vi "LINC Handshake Global.vi"(5 "target name":string, 7 "mode":T4, 8 "error in (no error)":errorcluster, 9 "handshake in":T1, 10 "command in":T2, 11 "GUID":string) -> (0 "error out":errorcluster, 1 "handshake out":T1, 2 "command out":T2, 3 "handshake":bool)   [LabVIEW 2018, in "STEPkgDriver_LINC.lvlib"]
uses:
  STEPkgDriver_LINC.lvlib
  LINC Command Origin.ctl
  LINC Command.ctl
  LINC Handshake Internal.ctl
  LINC Global Handshake Mode.ctl
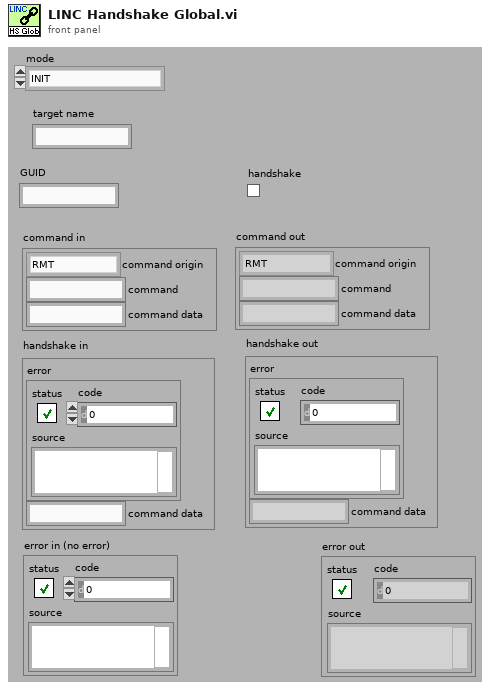
[diagram p1: front panel]
types:
  T1 = typedef "STEPkgDriver_LINC.lvlib/LINC Handshake Internal.ctl" = cluster{"error":errorcluster, "command data":string}
  T2 = typedef "STEPkgDriver_LINC.lvlib/LINC Command.ctl" = cluster{"command origin":T3, "command":string, "command data":string}
  T3 = typedef "STEPkgDriver_LINC.lvlib/LINC Command Origin.ctl" = enum8{"RMT", "LCL"}
  T4 = typedef "STEPkgDriver_LINC.lvlib/LINC Global Handshake Mode.ctl" = enum16{"INIT", "CLEAR", "ADD_COMMAND", "RMV_COMMAND", "CLR_HANDSHAKE", "SET_HANDSHAKE", "GET_HANDSHAKE"}
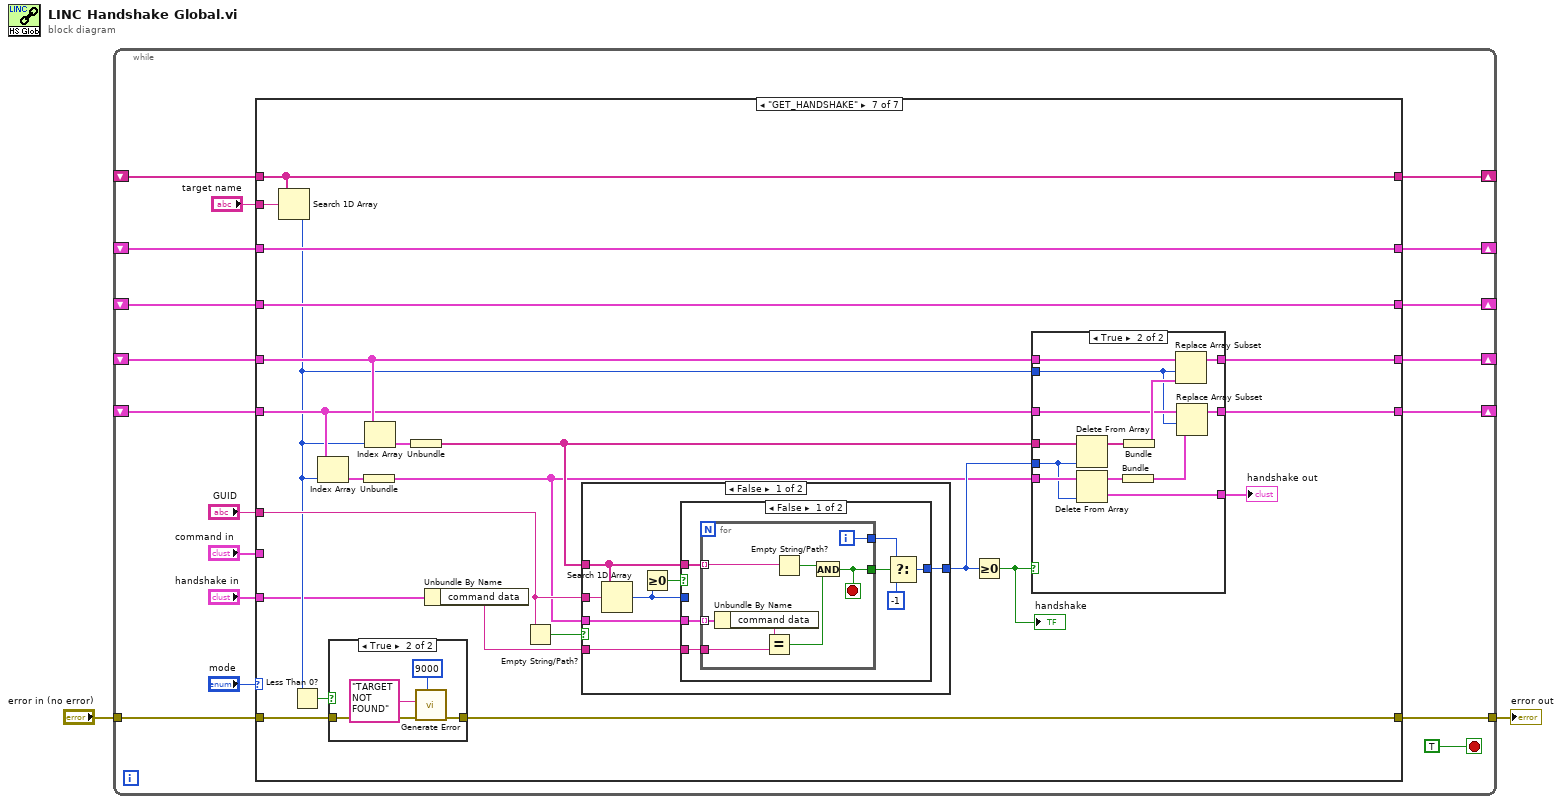
[diagram p0: block diagram]
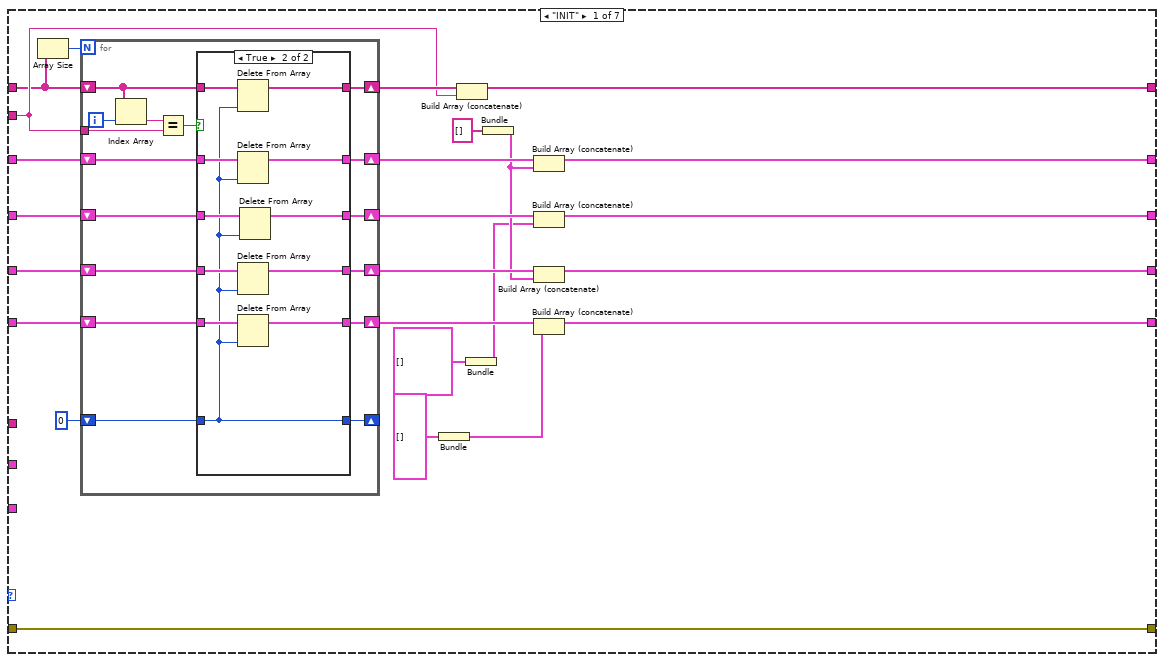
[diagram p2: hidden frame]
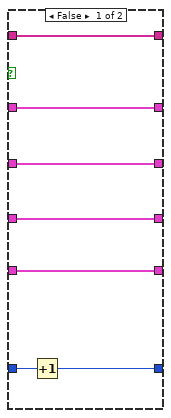
[diagram p3: hidden frame]
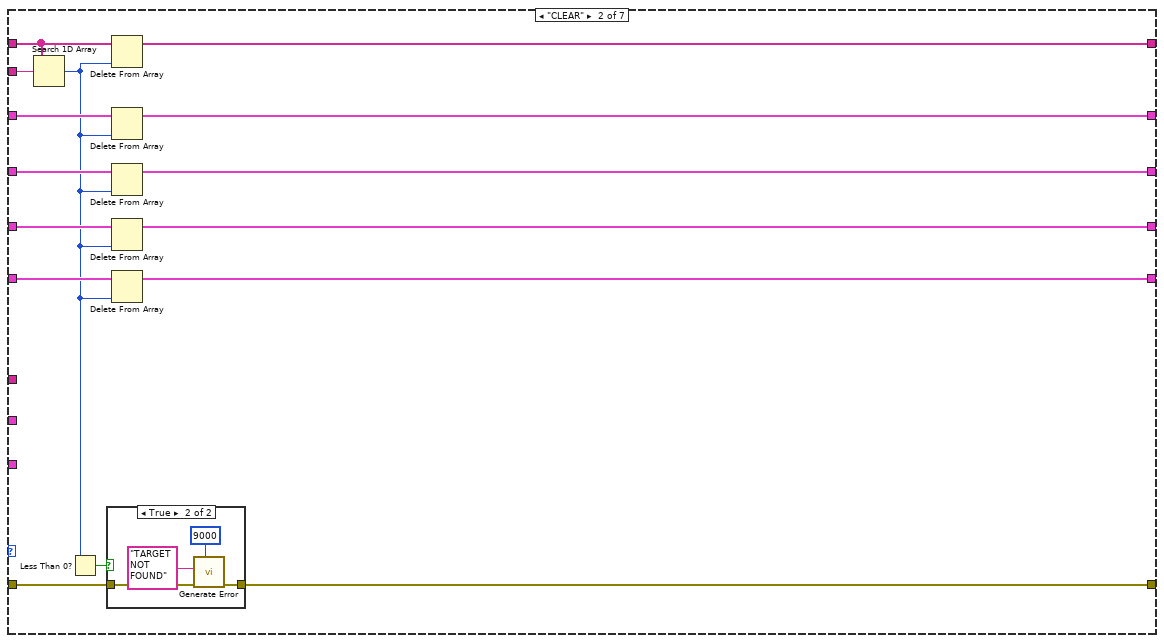
[diagram p4: hidden frame]
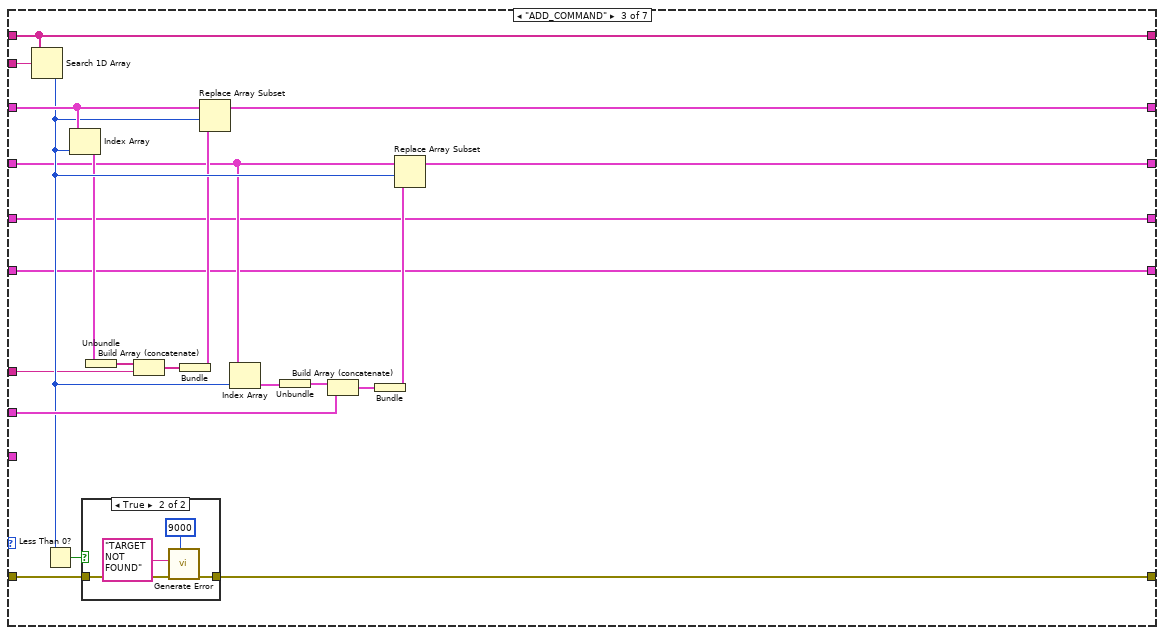
[diagram p6: hidden frame]
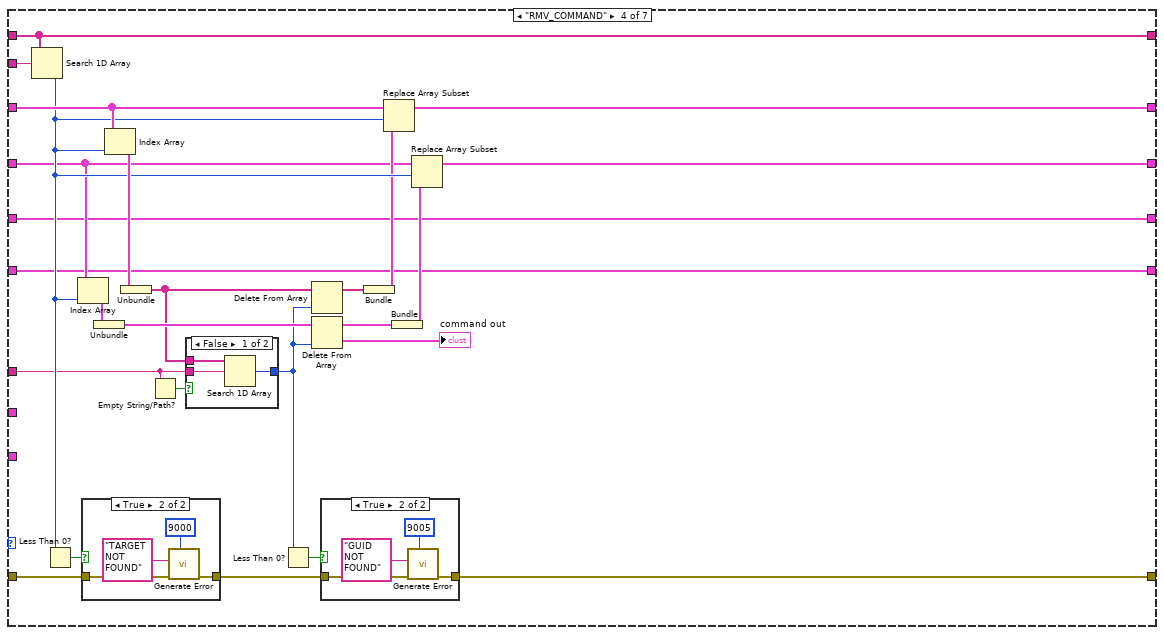
[diagram p8: hidden frame]
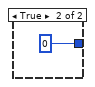
[diagram p9: hidden frame]
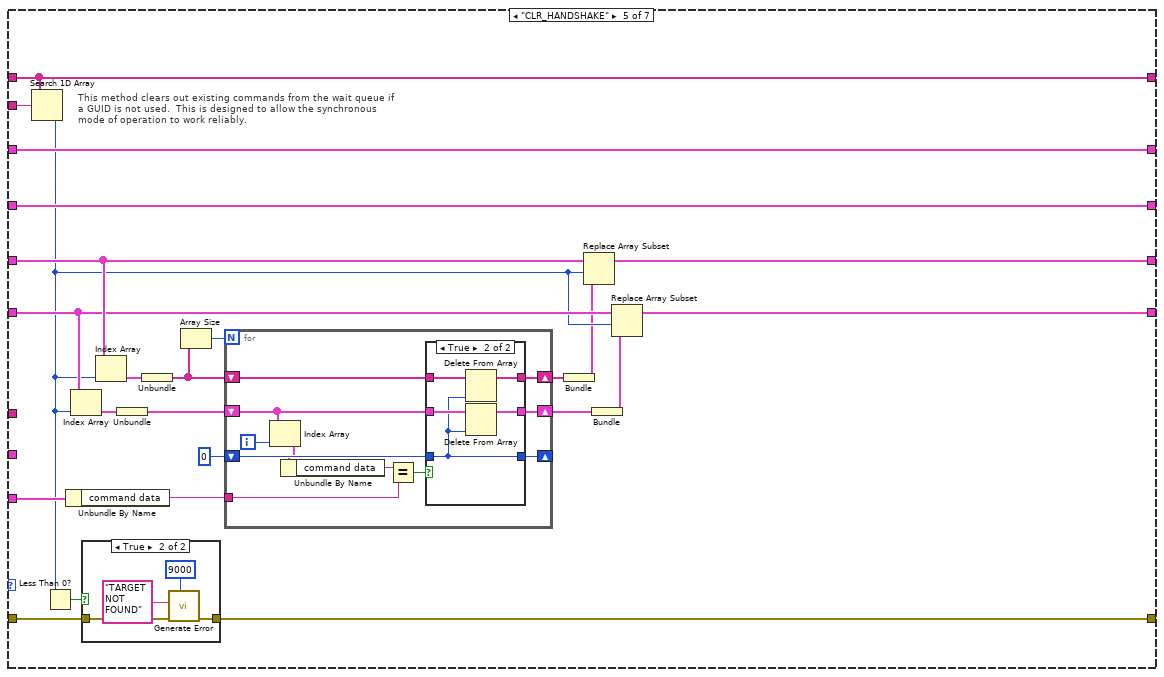
[diagram p12: hidden frame]
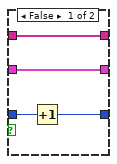
[diagram p13: hidden frame]
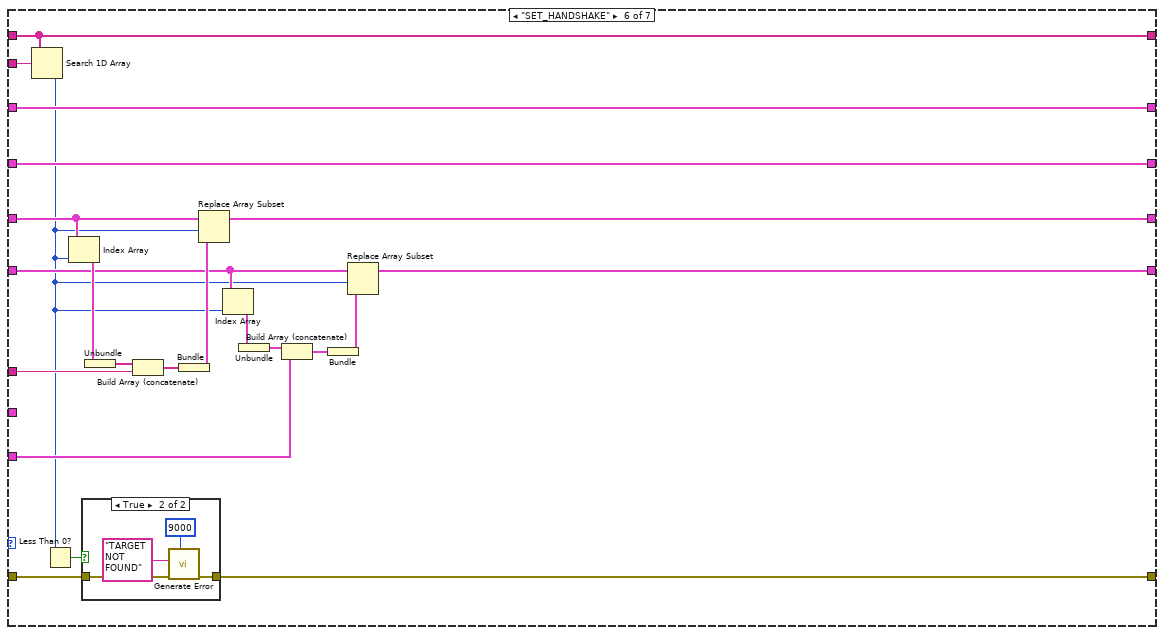
[diagram p15: hidden frame]
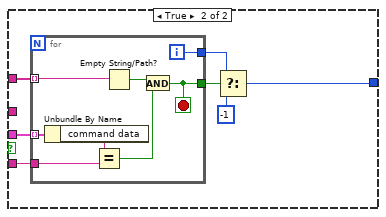
[diagram p19: hidden frame]
diagram:
  n1 = while {
    shift-right: [w18] -> _
    shift-left: _ -> [w19]
    tunnel: "error in (no error)" -> [w15]
    tunnel: [w14] -> w1
    shift-right: [w12] -> _
    shift-left: _ -> [w13]
    shift-right: [w10] -> _
    shift-left: _ -> [w9]
    shift-right: [w7] -> _
    shift-left: _ -> [w6]
    shift-right: [w5] -> _
    shift-left: _ -> [w4]
    stop <- TRUE stop-if-true
    n2 = case shown="\"GET_HANDSHAKE\"" "mode" {
      tunnel: w19 -> [w39 w93 w120 w151 w189 w236 w264]
      tunnel: [w45 w92 w120 w151 w189 w236 w264] -> w18
      tunnel: "target name" -> [w40 w94 w121 w152 w190 w237 w265]
      tunnel: w15 -> [w44 w90 w118 w149 w188 w234 w262]
      tunnel: [w44 w89 w117 w136 w186 w233 w256] -> w14
      tunnel: w13 -> [w41 w88 w101 w129 w184 w226 w252]
      tunnel: [w43 w87 w101 w129 w183 w225 w251] -> w12
      tunnel: "command in" -> [_ _ w114 _ _ _ _]
      tunnel: [w33 w85 w111 w147 w187 w227 w257] -> w10
      tunnel: w9 -> [w31 w86 w110 w148 w187 w227 w257]
      tunnel: "GUID" -> [_ _ w104 w133 _ w228 w259]
      tunnel: [w30 w83 w102 w131 w185 w224 w253] -> w7
      tunnel: w6 -> [w29 w84 w103 w130 w185 w224 w253]
      tunnel: w4 -> [w26 w82 w100 w128 w181 w222 w249]
      tunnel: [w25 w80 w100 w128 w182 w223 w250] -> w5
      tunnel: "handshake in" -> [_ _ _ _ w180 w217 w245]
      frame "INIT" {
        n3 = Array Size(array=w39) -> (size(s)=w38:i32)
        n4 = for {
          N: w38 -> [_]
          shift-right: [w55] -> w42
          shift-left: w39 -> [w60]
          shift-right: [w54] -> w36
          shift-left: w41 -> [w59]
          tunnel: w40 -> [w57]
          shift-right: [w52] -> _
          shift-left: 0 -> [w53]
          shift-right: [w50] -> w32
          shift-left: w31 -> [w51]
          shift-right: [w48] -> w28
          shift-left: w29 -> [w49]
          shift-right: [w47] -> w27
          shift-left: w26 -> [w46]
          i -> [w61]
          n5 = Index Array(array=w60, index=w61) -> (element=w58:string)
          n6 = Equal?(x=w58, y=w57) -> (x = y?=w56:bool)
          n7 = case shown="True" w56 {
            tunnel: w60 -> [w68 w79]
            tunnel: w59 -> [w67 w77]
            tunnel: [w68 w78] -> w55
            tunnel: [w67 w76] -> w54
            tunnel: w53 -> [w66 w69]
            tunnel: [w65 w69] -> w52
            tunnel: w51 -> [w64 w75]
            tunnel: [w64 w74] -> w50
            tunnel: w49 -> [w63 w73]
            tunnel: [w63 w72] -> w48
            tunnel: w46 -> [w62 w70]
            tunnel: [w62 w71] -> w47
            frame False {
              n8 = Increment(x=w66) -> (x+1=w65:i32)
            }
            frame True {
              n9 = Delete From Array(array=w79, index=w69) -> (array with subset deleted=w78:string[])  [unwired: 1 in, 1 out]
              n10 = Delete From Array(array=w75, index=w69) -> (array with subset deleted=w74:cluster{string[]}[])  [unwired: 1 in, 1 out]
              n11 = Delete From Array(array=w77, index=w69) -> (array with subset deleted=w76:cluster{string[]}[])  [unwired: 1 in, 1 out]
              n12 = Delete From Array(array=w70, index=w69) -> (array with subset deleted=w71:cluster{T1[]}[])  [unwired: 1 in, 1 out]
              n13 = Delete From Array(array=w73, index=w69) -> (array with subset deleted=w72:cluster{T2[]}[])  [unwired: 1 in, 1 out]
            }
          }
        }
        n14 = Bundle(T1[] []) -> (w21:cluster{T1[]})  [unwired: 1 in]
        n15 = Build Array (concatenate)(w42, w40) -> (w45:string[])
        n16 = Bundle(T2[] []) -> (w23:cluster{T2[]})  [unwired: 1 in]
        n17 = Bundle(string[] []) -> (w24:cluster{string[]})  [unwired: 1 in]
        n18 = Build Array (concatenate)(w32, w24) -> (w33:cluster{string[]}[])
        n19 = Build Array (concatenate)(w28, w23) -> (w30:cluster{T2[]}[])
        n20 = Build Array (concatenate)(w36, w24) -> (w43:cluster{string[]}[])
        n21 = Build Array (concatenate)(w27, w21) -> (w25:cluster{T1[]}[])
      }
      frame "CLEAR" {
        n22 = Search 1D Array(1D array=w93, element=w94) -> (index of element=w81:i32)  [unwired: 1 in]
        n23 = Less Than 0?(x=w81) -> (x < 0?=w91:bool)
        n24 = case shown="True" w91 {
          tunnel: w90 -> [w95 w99]
          tunnel: [w95 w98] -> w89
          frame False {
          }
          frame True {
            n25 = call "Generate Error.vi"("error code (-1301)"=9000, "error in"=w99, "description"="TARGET NOT FOUND") -> ("error out"=w98:errorcluster)  [unwired: 8 in]
          }
        }
        n26 = Delete From Array(array=w93, index=w81) -> (array with subset deleted=w92:string[])  [unwired: 1 in, 1 out]
        n27 = Delete From Array(array=w86, index=w81) -> (array with subset deleted=w85:cluster{string[]}[])  [unwired: 1 in, 1 out]
        n28 = Delete From Array(array=w84, index=w81) -> (array with subset deleted=w83:cluster{T2[]}[])  [unwired: 1 in, 1 out]
        n29 = Delete From Array(array=w88, index=w81) -> (array with subset deleted=w87:cluster{string[]}[])  [unwired: 1 in, 1 out]
        n30 = Delete From Array(array=w82, index=w81) -> (array with subset deleted=w80:cluster{T1[]}[])  [unwired: 1 in, 1 out]
      }
      frame "ADD_COMMAND" {
        n31 = Search 1D Array(1D array=w120, element=w121) -> (index of element=w109:i32)  [unwired: 1 in]
        n32 = Less Than 0?(x=w109) -> (x < 0?=w119:bool)
        n33 = Index Array(array=w110, index=w109) -> (element=w106:cluster{string[]})
        n34 = case shown="True" w119 {
          tunnel: w118 -> [w122 w126]
          tunnel: [w122 w125] -> w117
          frame False {
          }
          frame True {
            n35 = call "Generate Error.vi"("error code (-1301)"=9000, "error in"=w126, "description"="TARGET NOT FOUND") -> ("error out"=w125:errorcluster)  [unwired: 8 in]
          }
        }
        n36 = Unbundle(w106) -> (w107:string[])
        n37 = Build Array (concatenate)(w107, w104) -> (w108:string[])
        n38 = Bundle(w108) -> (w105:cluster{string[]})  [unwired: 1 in]
        n39 = Replace Array Subset(array=w110, new element=w105, index=w109) -> (w111:cluster{string[]}[])
        n40 = Index Array(array=w103, index=w109) -> (element=w116:cluster{T2[]})
        n41 = Unbundle(w116) -> (w115:T2[])
        n42 = Build Array (concatenate)(w115, w114) -> (w113:T2[])
        n43 = Bundle(w113) -> (w112:cluster{T2[]})  [unwired: 1 in]
        n44 = Replace Array Subset(array=w103, new element=w112, index=w109) -> (w102:cluster{T2[]}[])
      }
      frame "RMV_COMMAND" {
        n45 = Search 1D Array(1D array=w151, element=w152) -> (index of element=w144:i32)  [unwired: 1 in]
        n46 = Less Than 0?(x=w144) -> (x < 0?=w150:bool)
        n47 = Index Array(array=w130, index=w144) -> (element=w145:cluster{T2[]})
        n48 = case shown="True" w150 {
          tunnel: w149 -> [w162 w166]
          tunnel: [w162 w165] -> w137
          frame False {
          }
          frame True {
            n49 = call "Generate Error.vi"("error code (-1301)"=9000, "error in"=w166, "description"="TARGET NOT FOUND") -> ("error out"=w165:errorcluster)  [unwired: 8 in]
          }
        }
        n50 = Unbundle(w145) -> (w143:T2[])
        n51 = Index Array(array=w148, index=w144) -> (element=w146:cluster{string[]})
        n52 = Unbundle(w146) -> (w138:string[])
        n53 = Empty String/Path?(string/path=w133) -> (empty?=w132:bool)
        n54 = case shown="False" w132 {
          tunnel: w138 -> [w155 _]
          tunnel: w133 -> [w154 _]
          tunnel: [w153 0] -> w134
          frame False {
            n55 = Search 1D Array(1D array=w155, element=w154) -> (index of element=w153:i32)  [unwired: 1 in]
          }
          frame True {
          }
        }
        n56 = Less Than 0?(x=w134) -> (x < 0?=w135:bool)
        n57 = Delete From Array(array=w138, index=w134) -> (array with subset deleted=w142:string[])  [unwired: 1 in, 1 out]
        n58 = Delete From Array(array=w143, index=w134) -> (deleted portion=→"command out":T2, array with subset deleted=w140:T2[])  [unwired: 1 in]
        n59 = case shown="True" w135 {
          tunnel: w137 -> [w157 w161]
          tunnel: [w157 w160] -> w136
          frame False {
          }
          frame True {
            n60 = call "Generate Error.vi"("error code (-1301)"=9005, "error in"=w161, "description"="GUID NOT FOUND") -> ("error out"=w160:errorcluster)  [unwired: 8 in]
          }
        }
        n61 = Bundle(w142) -> (w141:cluster{string[]})  [unwired: 1 in]
        n62 = Replace Array Subset(array=w148, new element=w141, index=w144) -> (w147:cluster{string[]}[])
        n63 = Bundle(w140) -> (w139:cluster{T2[]})  [unwired: 1 in]
        n64 = Replace Array Subset(array=w130, new element=w139, index=w144) -> (w131:cluster{T2[]}[])
      }
      frame "CLR_HANDSHAKE" {
        # "This method clears out existing commands from the wait queue if a GUID is not used.  This is designed to allow the synchronous mode of operation to work reliably."
        n65 = Search 1D Array(1D array=w189, element=w190) -> (index of element=w176:i32)  [unwired: 1 in]
        n66 = Less Than 0?(x=w176) -> (x < 0?=w179:bool)
        n67 = Unbundle By Name(w180) -> ("command data"=w167:string)
        n68 = Index Array(array=w181, index=w176) -> (element=w177:cluster{T1[]})
        n69 = case shown="True" w179 {
          tunnel: w188 -> [w211 w215]
          tunnel: [w211 w214] -> w186
          frame False {
          }
          frame True {
            n70 = call "Generate Error.vi"("error code (-1301)"=9000, "error in"=w215, "description"="TARGET NOT FOUND") -> ("error out"=w214:errorcluster)  [unwired: 8 in]
          }
        }
        n71 = Index Array(array=w184, index=w176) -> (element=w178:cluster{string[]})
        n72 = Unbundle(w177) -> (w170:T1[])
        n73 = Unbundle(w178) -> (w169:string[])
        n74 = Array Size(array=w169) -> (size(s)=w168:i32)
        n75 = for {
          N: w168 -> [_]
          shift-right: [w200] -> w172
          shift-left: w169 -> [w201]
          shift-right: [w198] -> _
          shift-left: 0 -> [w199]
          shift-right: [w197] -> w171
          shift-left: w170 -> [w196]
          tunnel: w167 -> [w192]
          i -> [w195]
          n76 = Index Array(array=w196, index=w195) -> (element=w194:T1)
          n77 = Unbundle By Name(w194) -> ("command data"=w193:string)
          n78 = Equal?(x=w193, y=w192) -> (x = y?=w191:bool)
          n79 = case shown="True" w191 {
            tunnel: w201 -> [w205 w210]
            tunnel: [w205 w209] -> w200
            tunnel: w199 -> [w204 w206]
            tunnel: [w203 w206] -> w198
            tunnel: w196 -> [w202 w208]
            tunnel: [w202 w207] -> w197
            frame False {
              n80 = Increment(x=w204) -> (x+1=w203:i32)
            }
            frame True {
              n81 = Delete From Array(array=w210, index=w206) -> (array with subset deleted=w209:string[])  [unwired: 1 in, 1 out]
              n82 = Delete From Array(array=w208, index=w206) -> (array with subset deleted=w207:T1[])  [unwired: 1 in, 1 out]
            }
          }
        }
        n83 = Bundle(w172) -> (w175:cluster{string[]})  [unwired: 1 in]
        n84 = Replace Array Subset(array=w184, new element=w175, index=w176) -> (w183:cluster{string[]}[])
        n85 = Bundle(w171) -> (w174:cluster{T1[]})  [unwired: 1 in]
        n86 = Replace Array Subset(array=w181, new element=w174, index=w176) -> (w182:cluster{T1[]}[])
      }
      frame "SET_HANDSHAKE" {
        n87 = Search 1D Array(1D array=w236, element=w237) -> (index of element=w216:i32)  [unwired: 1 in]
        n88 = Less Than 0?(x=w216) -> (x < 0?=w235:bool)
        n89 = Index Array(array=w226, index=w216) -> (element=w230:cluster{string[]})
        n90 = case shown="True" w235 {
          tunnel: w234 -> [w238 w242]
          tunnel: [w238 w241] -> w233
          frame False {
          }
          frame True {
            n91 = call "Generate Error.vi"("error code (-1301)"=9000, "error in"=w242, "description"="TARGET NOT FOUND") -> ("error out"=w241:errorcluster)  [unwired: 8 in]
          }
        }
        n92 = Unbundle(w230) -> (w231:string[])
        n93 = Build Array (concatenate)(w231, w228) -> (w232:string[])
        n94 = Bundle(w232) -> (w229:cluster{string[]})  [unwired: 1 in]
        n95 = Replace Array Subset(array=w226, new element=w229, index=w216) -> (w225:cluster{string[]}[])
        n96 = Index Array(array=w222, index=w216) -> (element=w219:cluster{T1[]})
        n97 = Unbundle(w219) -> (w221:T1[])
        n98 = Build Array (concatenate)(w221, w217) -> (w220:T1[])
        n99 = Bundle(w220) -> (w218:cluster{T1[]})  [unwired: 1 in]
        n100 = Replace Array Subset(array=w222, new element=w218, index=w216) -> (w223:cluster{T1[]}[])
      }
      frame "GET_HANDSHAKE" {
        n101 = Search 1D Array(1D array=w264, element=w265) -> (index of element=w247:i32)  [unwired: 1 in]
        n102 = Less Than 0?(x=w247) -> (x < 0?=w263:bool)
        n103 = Index Array(array=w249, index=w247) -> (element=w248:cluster{T1[]})
        n104 = case shown="True" w263 {
          tunnel: w262 -> [w319 w323]
          tunnel: [w319 w322] -> w256
          frame False {
          }
          frame True {
            n105 = call "Generate Error.vi"("error code (-1301)"=9000, "error in"=w323, "description"="TARGET NOT FOUND") -> ("error out"=w322:errorcluster)  [unwired: 8 in]
          }
        }
        n106 = Unbundle(w248) -> (w243:T1[])
        n107 = Index Array(array=w252, index=w247) -> (element=w261:cluster{string[]})
        n108 = Unbundle(w261) -> (w260:string[])
        n109 = Unbundle By Name(w245) -> ("command data"=w246:string)
        n110 = Empty String/Path?(string/path=w259) -> (empty?=w258:bool)
        n111 = case shown="False" w258 {
          tunnel: w260 -> [w283 w306]
          tunnel: w259 -> [w287 _]
          tunnel: [w284 w307] -> w255
          tunnel: w243 -> [w282 w305]
          tunnel: w246 -> [w281 w304]
          frame False {
            n112 = Search 1D Array(1D array=w283, element=w287) -> (index of element=w285:i32)  [unwired: 1 in]
            n113 = Greater Or Equal To 0?(x=w285) -> (x >= 0?=w286:bool)
            n114 = case shown="False" w286 {
              tunnel: w285 -> [_ w303]
              tunnel: [w288 w303] -> w284
              tunnel: w283 -> [w294 _]
              tunnel: w282 -> [w293 _]
              tunnel: w281 -> [w292 _]
              frame False {
                n115 = for {
                  tunnel: w294 -> [w301] mode=indexing
                  tunnel: w293 -> [w296] mode=indexing
                  tunnel: w292 -> [w302]
                  tunnel: [w298] -> w291
                  tunnel: [w297] -> w290
                  i -> [w297]
                  stop <- w298 stop-if-true
                  n116 = Unbundle By Name(w296) -> ("command data"=w295:string)
                  n117 = Equal?(x=w295, y=w302) -> (x = y?=w299:bool)
                  n118 = Empty String/Path?(string/path=w301) -> (empty?=w300:bool)
                  n119 = And(x=w300, y=w299) -> (x .and. y?=w298:bool)
                }
                n120 = Select(t=w290, s=w291, f=-1) -> (s? t:f=w288:i32)
              }
              frame True {
              }
            }
          }
          frame True {
            n121 = for {
              tunnel: w306 -> [w317] mode=indexing
              tunnel: w305 -> [w312] mode=indexing
              tunnel: w304 -> [w318]
              tunnel: [w314] -> w310
              tunnel: [w313] -> w308
              i -> [w313]
              stop <- w314 stop-if-true
              n122 = Unbundle By Name(w312) -> ("command data"=w311:string)
              n123 = Equal?(x=w311, y=w318) -> (x = y?=w315:bool)
              n124 = Empty String/Path?(string/path=w317) -> (empty?=w316:bool)
              n125 = And(x=w316, y=w315) -> (x .and. y?=w314:bool)
            }
            n126 = Select(t=w308, s=w310, f=-1) -> (s? t:f=w307:i32)
          }
        }
        n127 = Greater Or Equal To 0?(x=w255) -> (x >= 0?=w254:bool)
        "handshake" <- w254
        n128 = case shown="True" w254 {
          tunnel: w247 -> [_ w273]
          tunnel: w260 -> [_ w278]
          tunnel: w255 -> [_ w271]
          tunnel: w252 -> [w267 w277]
          tunnel: [w267 w276] -> w251
          tunnel: w249 -> [w266 w275]
          tunnel: [w266 w274] -> w250
          tunnel: w243 -> [_ w272]
          tunnel: [_ w268] -> w244
          frame False {
          }
          frame True {
            n129 = Delete From Array(array=w278, index=w271) -> (array with subset deleted=w280:string[])  [unwired: 1 in, 1 out]
            n130 = Delete From Array(array=w272, index=w271) -> (deleted portion=w268:T1, array with subset deleted=w270:T1[])  [unwired: 1 in]
            n131 = Bundle(w270) -> (w269:cluster{T1[]})  [unwired: 1 in]
            n132 = Bundle(w280) -> (w279:cluster{string[]})  [unwired: 1 in]
            n133 = Replace Array Subset(array=w277, new element=w279, index=w273) -> (w276:cluster{string[]}[])
            n134 = Replace Array Subset(array=w275, new element=w269, index=w273) -> (w274:cluster{T1[]}[])
          }
        }
        "handshake out" <- w244
      }
    }
  }
  "error out" <- w1
